vi "boolean_odd_even_enumeration.vi"() -> ()   [LabVIEW 2019]
panel:
  in  "btn3":bool
  in  "btn2":bool
  in  "btn1":bool
  out "Even?":bool
  in  "Numeric":i32
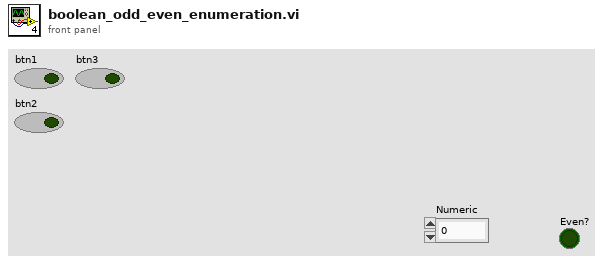
[diagram p1: front panel]
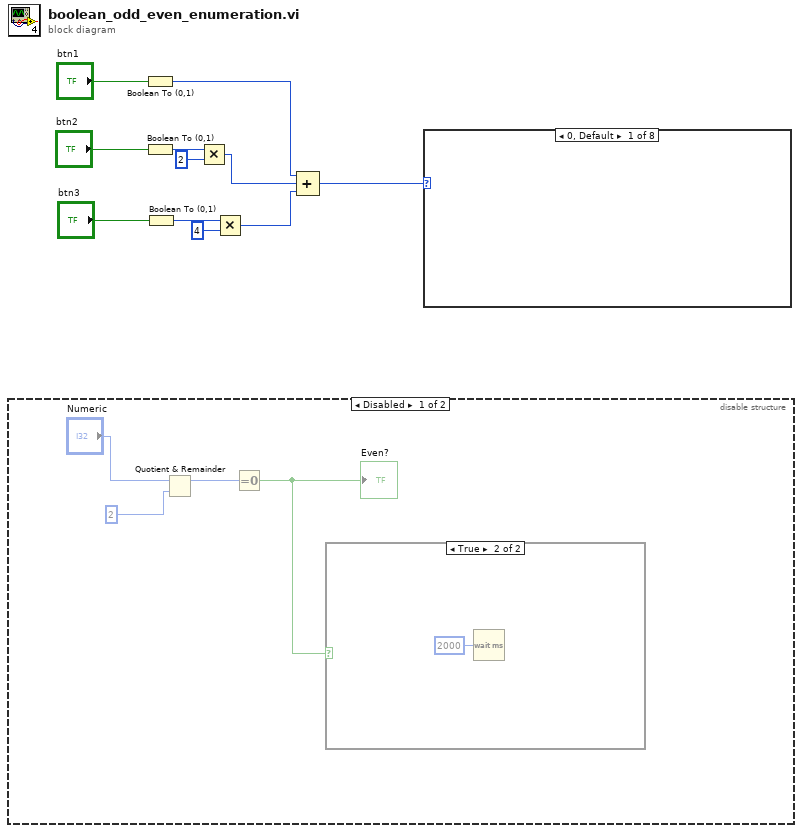
[diagram p0: block diagram]
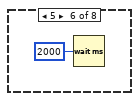
[diagram p8: hidden frame]
diagram:
  n1 = disable-structure shown="Disabled" {
    frame Disabled {
      n2 = Quotient & Remainder(x="Numeric", y=2) -> (x-y*floor(x/y)=w13:i32)  [unwired: 1 out]
      n3 = Equal To 0?(x=w13) -> (x = 0?=w12:bool)
      "Even?" <- w12
      n4 = case shown="True" w12 {
        frame False {
        }
        frame True {
          n5 = Wait (ms)(milliseconds to wait=u32 2000) -> ()  [unwired: 1 out]
        }
      }
    }
    frame Enabled {
    }
  }
  n6 = Boolean To (0,1)(Boolean="btn1") -> (0, 1=w4:i16)
  n7 = Boolean To (0,1)(Boolean="btn2") -> (0, 1=w8:i16)
  n8 = Boolean To (0,1)(Boolean="btn3") -> (0, 1=w5:i16)
  n9 = Multiply(x=w8, y=i16 2) -> (x*y=w3:i16)
  n10 = Multiply(x=w5, y=i16 4) -> (x*y=w2:i16)
  n11 = Compound Arithmetic op=ADD(w4, w3, w2) -> (w1:i16)
  n12 = case shown="0, Default" w1 {
    frame 0, Default {
    }
    frame 1 {
    }
    frame 2 {
    }
    frame 3 {
    }
    frame 4 {
    }
    frame 5 {
      n13 = Wait (ms)(milliseconds to wait=u32 2000) -> ()  [unwired: 1 out]
    }
    frame 6 {
    }
    frame 7 {
    }
  }
